vi "lib Matchpattern to Array of String.vi"(8 "error in (no error)":errorcluster, 10 "filenames":string[](array[string]), 11 "Pattern":string) -> (0 "error out":errorcluster, 3 "Matches":string[](array[string]))   [LabVIEW 2016]
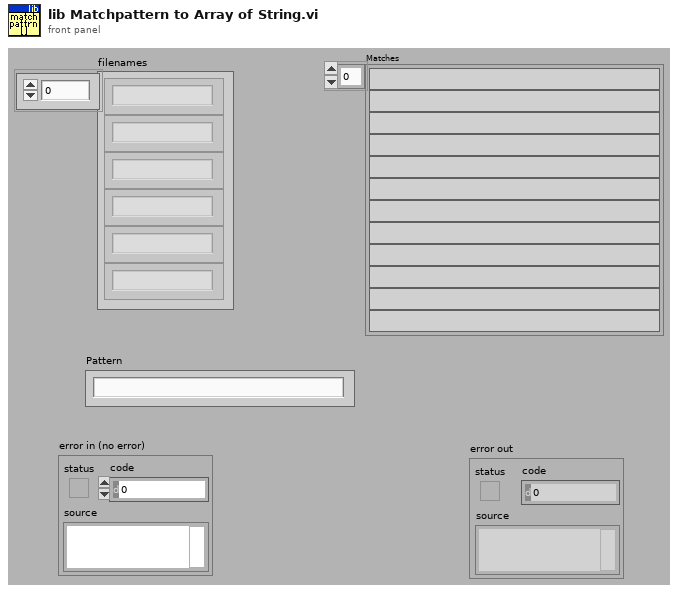
[diagram p1: front panel]
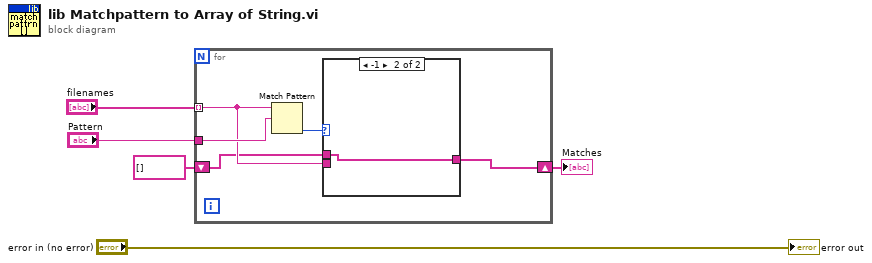
[diagram p0: block diagram]
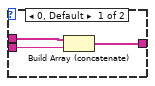
[diagram p2: hidden frame]
diagram:
  n1 = for {
    tunnel: "filenames" -> [w8] mode=indexing
    tunnel: "Pattern" -> [w10]
    shift-right: [w7] -> w1
    shift-left: string[] [] -> [w6]
    n2 = Match Pattern(string=w8, regular expression=w10) -> (offset past match=w9:i32)  [unwired: 1 in, 3 out]
    n3 = case shown="-1" w9 {
      tunnel: w8 -> [w13 _]
      tunnel: [w12 w14] -> w7
      tunnel: w6 -> [w11 w14]
      frame 0, Default {
        n4 = Build Array (concatenate)(w11, w13) -> (w12:string[])
      }
      frame -1 {
      }
    }
  }
  "Matches" <- w1
  "error out" <- "error in (no error)"
